vi "Initialize.vi"(8 "error in (no error)":errorcluster, 9 "Process Gain":dbl, 10 "Time Constant":dbl, 11 "Process Simulator in":refnum<class "Process Simulator.lvclass">) -> (0 "error out":errorcluster, 3 "Process Simulator out":refnum<class "Process Simulator.lvclass">)   [LabVIEW 2024, in "PID.lvlib" / "Process Simulator.lvclass"]
uses:
  Process Simulator.lvclass
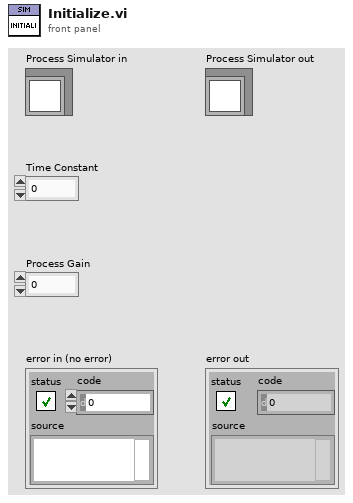
[diagram p1: front panel]
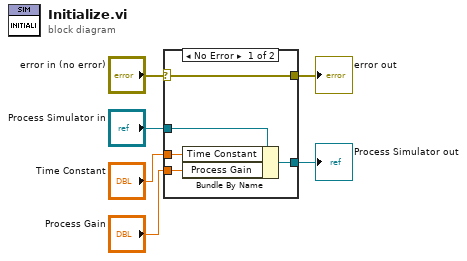
[diagram p0: block diagram]
diagram:
  n1 = case shown="No Error" "error in (no error)" {
    selector: "error in (no error)" -> [w11 w13]
    tunnel: [w11 w13] -> w5
    tunnel: [w7 w12] -> w3
    tunnel: "Process Simulator in" -> [w10 w12]
    tunnel: "Time Constant" -> [w9 _]
    tunnel: "Process Gain" -> [w8 _]
    frame No Error {
      n2 = Bundle By Name(cluster=w10, "Time Constant"=w9, "Process Gain"=w8) -> (w7:refnum<class "Process Simulator.lvclass">)
    }
    frame Error {
    }
  }
  "error out" <- w5
  "Process Simulator out" <- w3
